vi "Log.vi"(10 "Log Packet":T1, 11 "SystemLog Sink in":refnum<class "SystemLog Sink.lvclass">) -> (0 "error out":errorcluster, 3 "SystemLog Sink out":refnum<class "SystemLog Sink.lvclass">)   [LabVIEW 2017, in "SystemLog Sink.lvclass"]
uses:
  <vilib>/gpm_packages/@cs/event-logger/Source/SystemLog Sink/SystemLog Sink.lvclass
  C:/Program Files/National Instruments/LabVIEW 2017/vi.lib/gpm_packages/@cs/event-logger/Source/String Log Sink/String Log Sink.lvclass
  <vilib>/gpm_packages/@cs/event-logger/Source/Composed Log/Types/Log Packet.ctl
  <vilib>/gpm_packages/@cs/event-logger/Source/Composed Log/Types/Log Level.ctl
  <vilib>/gpm_packages/@cs/event-logger/Source/String Log Sink/String Log Sink.lvclass/String Log Sink.ctl
  <vilib>/gpm_packages/@cs/event-logger/Source/IStringFormat/IStringFormat.lvclass
  <vilib>/Utility/SystemLogging/NI_SystemLogging.lvlib
  <vilib>/gpm_packages/@cs/event-logger/Source/String Log Sink/String Log Sink.lvclass
  <vilib>/gpm_packages/@cs/event-logger/Source/Composed Log/Composed Log.lvlib
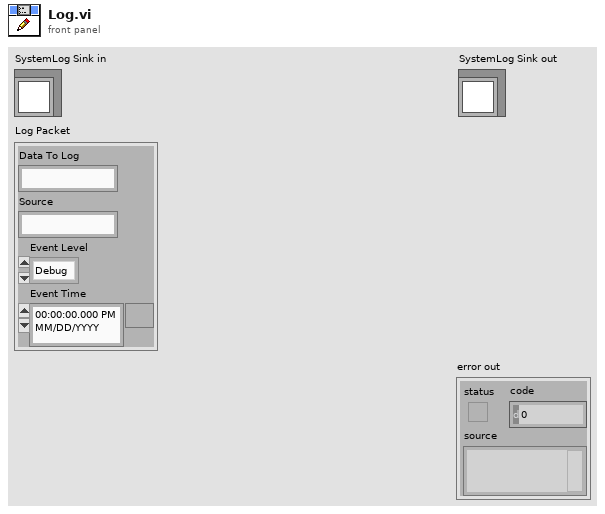
[diagram p1: front panel]
types:
  T1 = typedef "Composed Log.lvlib/Log Packet.ctl" = cluster{"Data To Log":string, "Source":string, "Event Level":T2, "Event Time":timestamp}
  T2 = typedef "Composed Log.lvlib/Log Level.ctl" = enum16{"Debug", "Info", "Warning", "Error", "Critical"}
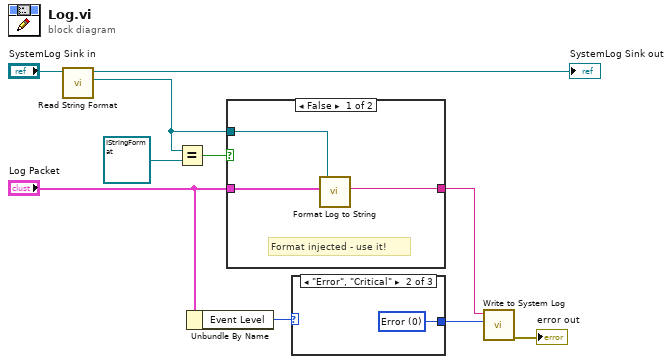
[diagram p0: block diagram]
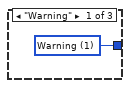
[diagram p2: hidden frame]
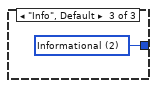
[diagram p3: hidden frame]
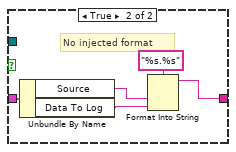
[diagram p4: hidden frame]
diagram:
  n1 = call <vilib>:"Read String Format.vi"("String Log Sink in"="SystemLog Sink in") -> ("String Format"=w1:refnum<class "IStringFormat.lvclass">, "String Log Sink out"=→"SystemLog Sink out":refnum<class "SystemLog Sink.lvclass">)  [unwired: 8 in, 1 out]
  n2 = Equal?(x=w1, y=refnum<class "IStringFormat.lvclass"> refnum) -> (x = y?=w9:bool)
  n3 = Unbundle By Name("Log Packet") -> ("Event Level"=w7:T2)
  n4 = case shown="False" w9 {
    tunnel: w1 -> [w13 _]
    tunnel: "Log Packet" -> [w12 w18]
    tunnel: [w11 w14] -> w5
    frame False {
      # "Format injected - use it!"
      n5 = call-dynamic "Format Log to String.vi"("Log Packet"=w12, "IStringFormat in"=w13) -> ("Log Entry"=w11:string)  [unwired: 8 in, 1 out]
    }
    frame True {
      # "No injected format"
      n6 = Unbundle By Name(w18) -> ("Source"=w17:string, "Data To Log"=w16:string)
      n7 = Format Into String(format string="%s.%s", w17, w16) -> (resulting string=w14:string)  [unwired: 2 in, 1 out]
    }
  }
  n8 = case shown="\"Error\", \"Critical\"" w7 {
    tunnel: [w19 w20 w21] -> w6
    frame "Warning" {
      w19 = 1 items=["Error", "Warning", "Informational"] ("severity")
    }
    frame "Error", "Critical" {
      w20 = 0 items=["Error", "Warning", "Informational"] ("severity")
    }
    frame "Info", Default {
      w21 = 2 items=["Error", "Warning", "Informational"] ("severity")
    }
  }
  n9 = call <vilib>:"Write to System Log.vi"("severity"=w6, "message"=w5) -> ("error out"=→"error out":errorcluster)  [unwired: 9 in]
